vi "Read Measurement (ASK Demodulation).vi"(0 "VISA resource name":refnum<visa-resource-name>, 11 "error in (no error)":errorcluster) -> (3 "ASK Depth (%)":dbl[](array[numeric]), 4 "VISA resource name out":refnum<visa-resource-name>, 6 "ASK Error (%)":dbl[](array[numeric]), 8 "ASK Index (%)":dbl[](array[numeric]), 10 "Carrier Power (dBm)":dbl[](array[numeric]), 14 "Carrier Frequency Offset (Hz)":dbl[](array[numeric]), 15 "error out":errorcluster)   [LabVIEW 2022 SP3, in "Agilent N934X Series.lvlib"]
doc: "Reads the measurement result from the spectrum analyzer(ASK Demodulation Measurement).\n\nNotes:\n\n(1) This VI is only available for N9321C, N9322C, N9323C, N9324C models.\n(2) User must use <B>Configure Measurement Type.vi</B> to change the mode to <B>ASK Modulation</B> before using this VI."
uses:
  <instrlib>/Agilent N934X Series/Agilent N934X Series.lvlib
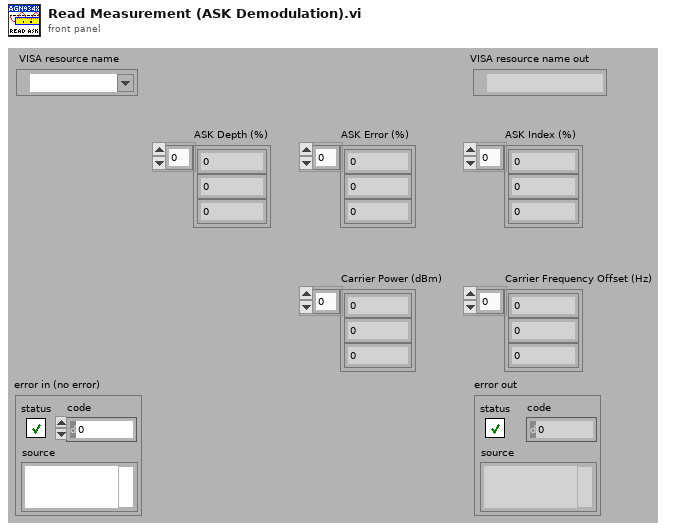
[diagram p1: front panel]
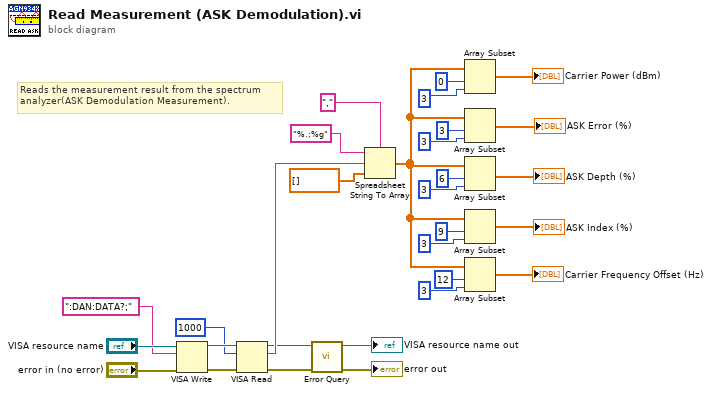
[diagram p0: block diagram]
diagram:
  # "Reads the measurement result from the spectrum\nanalyzer(ASK Demodulation Measurement)."
  n1 = VISA Write(VISA resource name="VISA resource name", write buffer=":DAN:DATA?;", error in (no error)="error in (no error)") -> (VISA resource name out=w29:refnum<visa-resource-name>, error out=w30:errorcluster)  [unwired: 1 out]
  n2 = VISA Read(VISA resource name=w29, byte count=u32 1000, error in (no error)=w30) -> (VISA resource name out=w2:refnum<visa-resource-name>, read buffer=w21:string, error out=w3:errorcluster)  [unwired: 1 out]
  n3 = call <instrlib>:"Error Query.vi"("error in (no error)"=w3, "VISA resource name"=w2) -> ("error out"=→"error out":errorcluster, "VISA resource name out"=→"VISA resource name out":refnum<visa-resource-name>)  [unwired: 6 in, 2 out]
  n4 = Spreadsheet String To Array(delimiter (Tab)=",", format string="%.;%g", spreadsheet string=w21, array type (2D Dbl)=dbl[] [] ("Measurement Data 2")) -> (array=w1:dbl[])
  n5 = Array Subset(array=w1, index=0, length=3) -> (→"Carrier Power (dBm)":dbl[])
  n6 = Array Subset(array=w1, index=3, length=3) -> (→"ASK Error (%)":dbl[])
  n7 = Array Subset(array=w1, index=6, length=3) -> (→"ASK Depth (%)":dbl[])
  n8 = Array Subset(array=w1, index=9, length=3) -> (→"ASK Index (%)":dbl[])
  n9 = Array Subset(array=w1, index=12, length=3) -> (→"Carrier Frequency Offset (Hz)":dbl[])
